vi "set_alarm_TPG361.vi"(6 "cluster_ref_TPG361":T1, 8 "time_last_audio_alarm_in":timestamp, 10 "warning":bool, 11 "error":bool) -> (0 "time_last_audio_alarm_out":timestamp)   [LabVIEW 2019]
uses:
  cluster_ref_TPG361.ctl
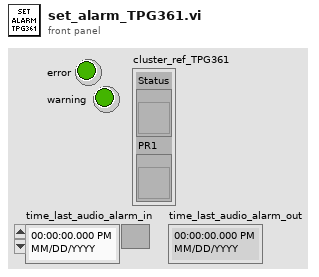
[diagram p1: front panel]
types:
  T1 = typedef "cluster_ref_TPG361.ctl" = cluster{"Status":refnum<vi>, "PR1":refnum<vi>}
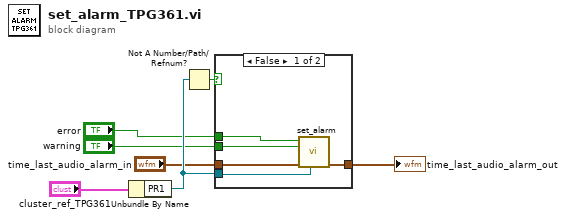
[diagram p0: block diagram]
diagram:
  n1 = Unbundle By Name("cluster_ref_TPG361") -> ("PR1"=w5:refnum<vi>)
  n2 = Not A Number/Path/Refnum?(number/path/refnum=w5) -> (NaN/Path/Refnum?=w7:bool)
  n3 = case shown="False" w7 {
    tunnel: w5 -> [w12 _]
    tunnel: "error" -> [w11 _]
    tunnel: "warning" -> [w10 _]
    tunnel: [w9 w13] -> w2
    tunnel: "time_last_audio_alarm_in" -> [w8 w13]
    frame False {
      n4 = call "set_alarm.vi"("value_ref"=w12, "time_last_audio_alarm_in"=w8, "warning"=w10, "error"=w11) -> ("time_last_audio_alarm_out"=w9:timestamp)  [unwired: 7 in]
    }
    frame True {
    }
  }
  "time_last_audio_alarm_out" <- w2
